vi "CODMn通讯.vi"() -> ()   [LabVIEW 2016]
uses:
  <vilib>/Plasmionique/MB Master/MB Master.lvlib
  <vilib>/Utility/config.llb/NI_LVConfig.lvlib
panel:
  in  "读取数据":bool
  in  "释放串口":bool
  in  "打开串口":bool
  out "队列中元素数量":i32
  out "元素":cluster{"命令":string}[](array[cluster])
  out "待处理插入数量":i32
  out "读取公式":u16[](array[numeric])
  out "读取参数":u16[](array[numeric])
  out "数据存储":u16[](array[numeric])
  out "温度":bool[](array[boolean])
  out "M输出点":bool[](array[boolean])
  out "ORP、时间":u16[](array[numeric])
  out "测量状态":u16[](array[numeric])
  out "通讯状态":bool
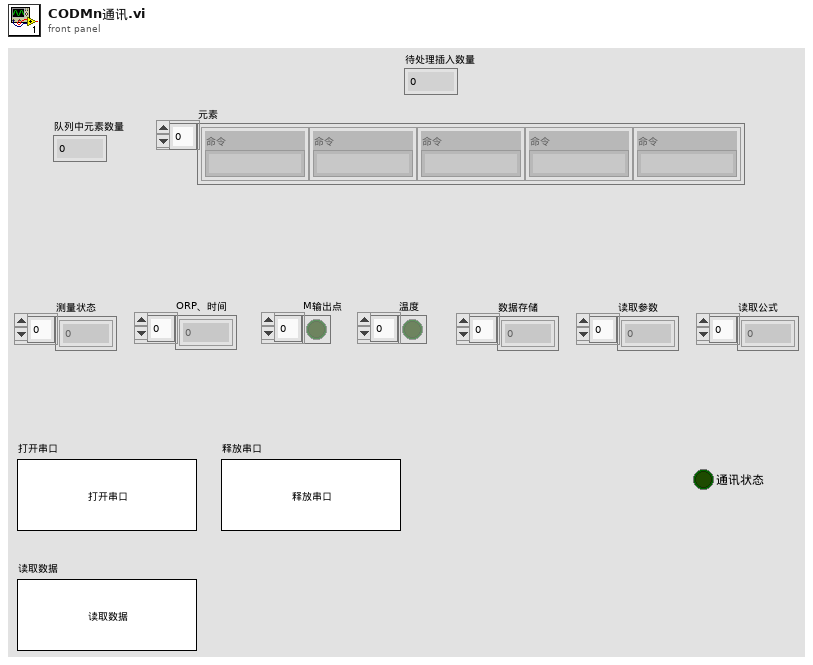
[diagram p1: front panel]
types:
  T1 = typedef "NI_LVConfig.lvlib/Config Data RefNum.ctl" = refnum<k1>
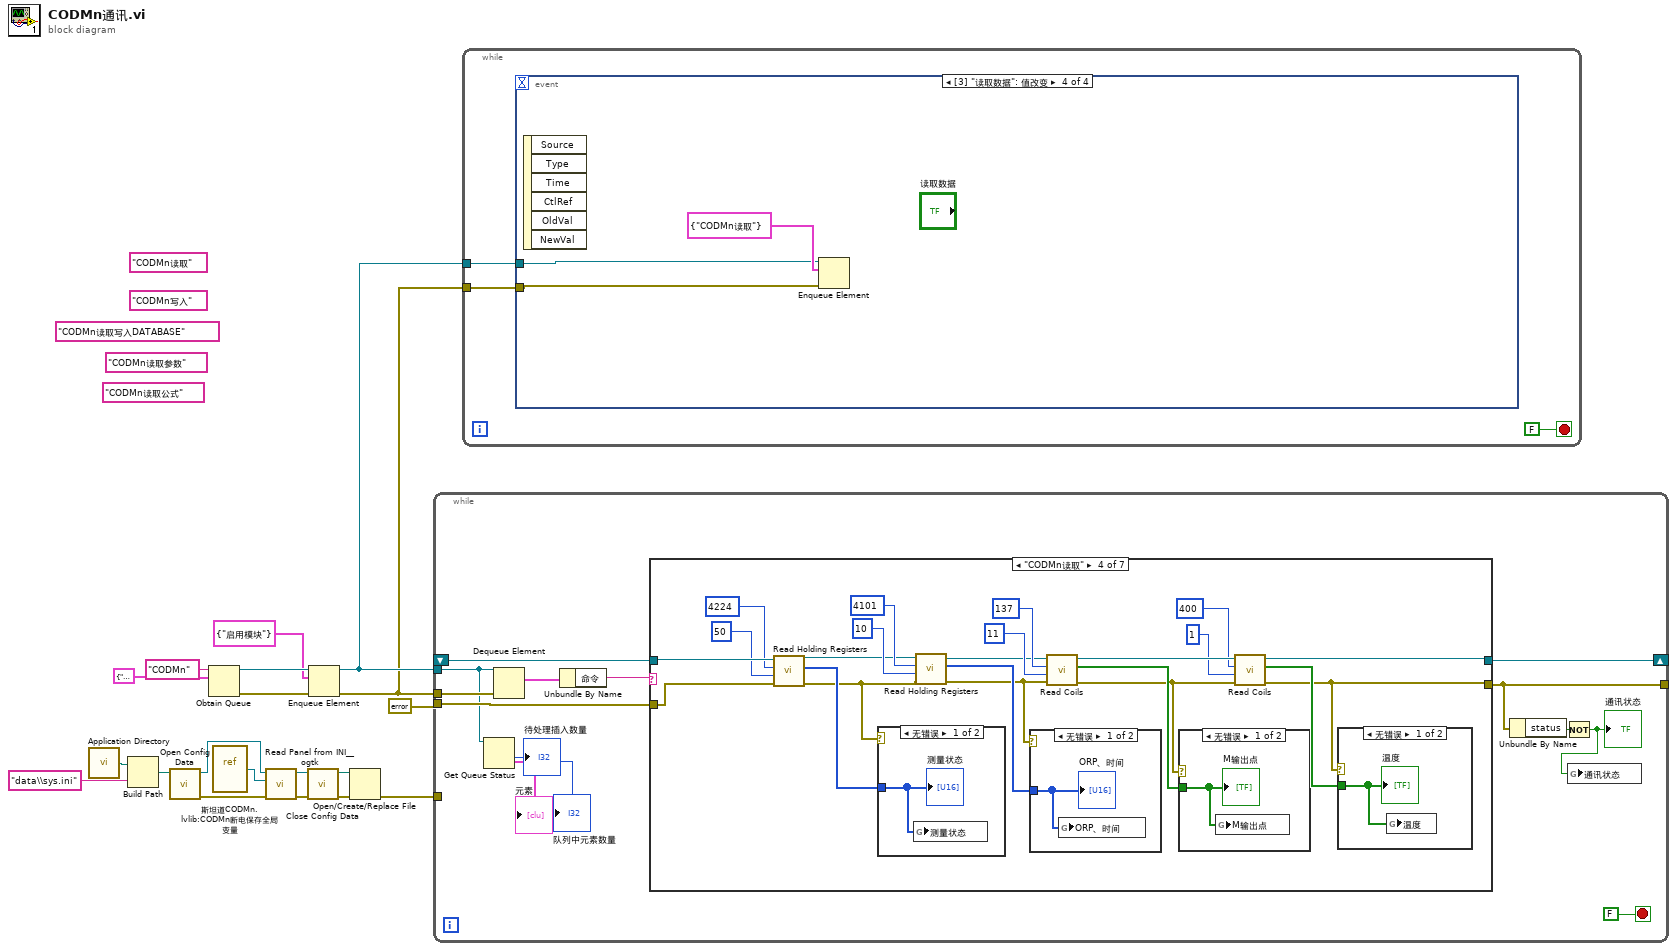
[diagram p0: block diagram]
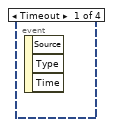
[diagram p2: hidden frame]
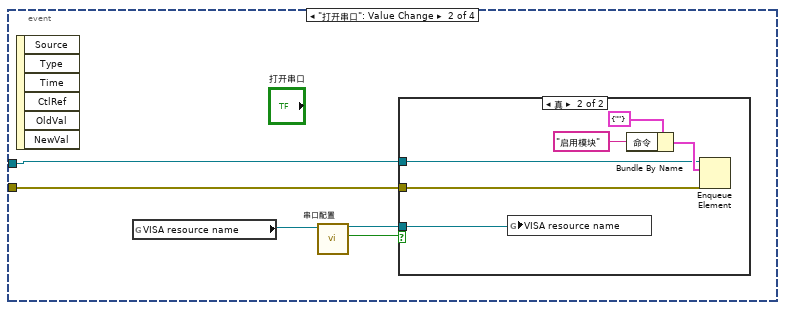
[diagram p3: hidden frame]
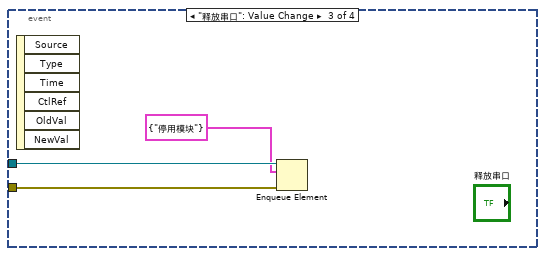
[diagram p5: hidden frame]
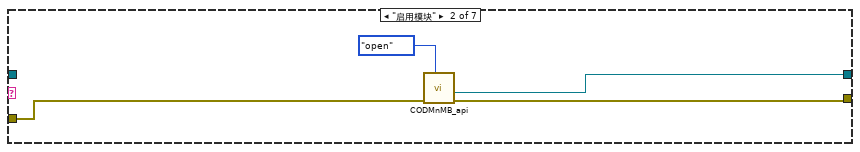
[diagram p7: hidden frame]
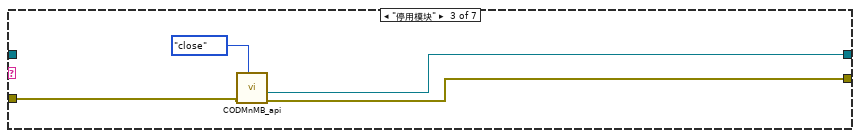
[diagram p8: hidden frame]
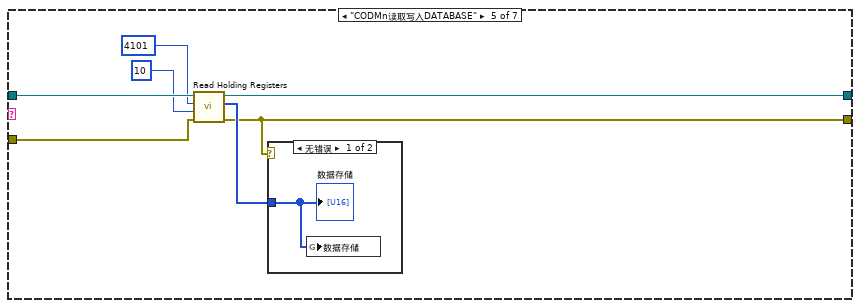
[diagram p13: hidden frame]
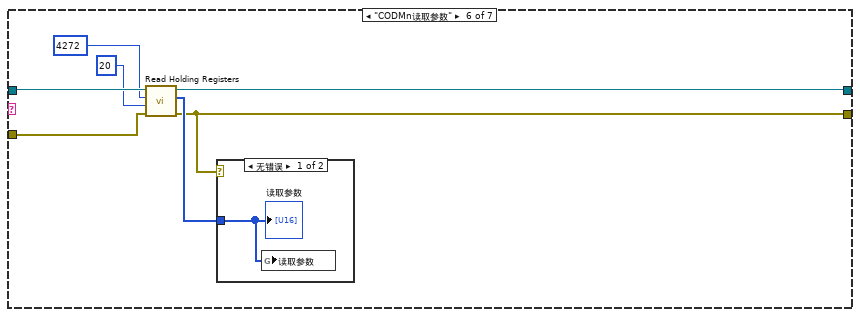
[diagram p15: hidden frame]
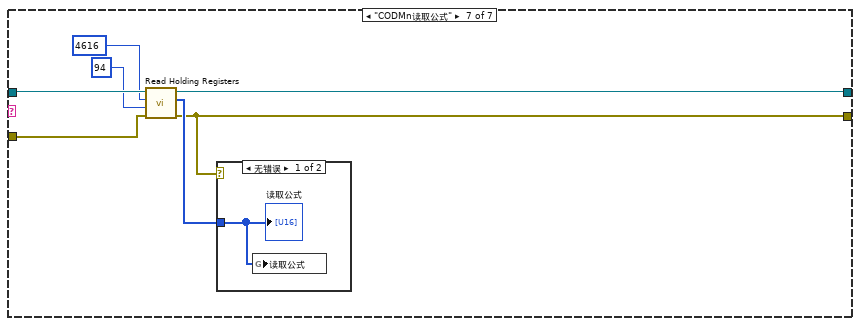
[diagram p17: hidden frame]
diagram:
  (unwired) "CODMn读取公式" ("名称（未命名）")
  (unwired) "CODMn读取写入DATABASE" ("名称（未命名）")
  (unwired) "CODMn读取参数" ("名称（未命名）")
  (unwired) "CODMn读取" ("名称（未命名）")
  (unwired) "CODMn写入" ("名称（未命名）")
  n1 = call <vilib>:"Application Directory.vi"() -> ("Application Directory"=w13:path)
  n2 = Build Path(base path=w13, name or relative path="data\\sys.ini" ("名称或相对路径")) -> (appended path=w11:path)
  n3 = call <vilib>:"Open Config Data.vi"("configuration file path"=w11) -> ("error out"=w7:errorcluster, "refnum"=w10:T1)  [unwired: 8 in, 1 out]
  n4 = Obtain Queue(name (unnamed)="CODMn" ("名称（未命名）"), element data type=cluster{"命令":string} {"命令"="启用模块"} ("元素")) -> (queue out=w16:refnum<queue>, error out=w15:errorcluster)  [unwired: 3 in, 1 out]
  n5 = vi-ref "斯坦道CODMn.lvlib:CODMn断电保存全局变量.vi"() -> (w9:refnum<vi>)
  n6 = call <userlib>:"Read Panel from INI__ogtk.vi"("error in (no error)"=w7, "VI ref"=w9, "refnum"=w10) -> ("error out"=w6:errorcluster, "refnum out"=w8:T1)  [unwired: 7 in]
  n7 = call <vilib>:"Close Config Data.vi"("error in (no error)"=w6, "refnum"=w8) -> ("error out"=w5:errorcluster, "file path"=w4:path)  [unwired: 8 in]
  n8 = Enqueue Element(queue=w16, element=cluster{"命令":string} {"命令"="启用模块"} ("元素"), error in (no error)=w15) -> (queue out=w2:refnum<queue>, error out=w1:errorcluster)  [unwired: 1 in, 1 out]
  n9 = Open/Create/Replace File(file path (use dialog)=w4, error in=w5) -> (error out=w3:errorcluster)  [unwired: 4 in, 2 out]
  n10 = while {
    tunnel: w2 -> [w23]
    tunnel: w1 -> [w32]
    tunnel: [w24] -> _
    shift-right: [w28] -> _
    shift-left: _ -> [w27]
    tunnel: errorcluster {"status"=FALSE, "code"=0, "source"=""} ("error out") -> [w26]
    tunnel: w3 -> [_]
    stop <- FALSE stop-if-true
    n11 = Get Queue Status(queue=w23) -> (# pending insert=→"待处理插入数量":i32, # elements in queue=→"队列中元素数量":i32, elements=→"元素":cluster{"命令":string}[])  [unwired: 2 in, 5 out]
    n12 = Dequeue Element(queue=w23, error in (no error)=w32) -> (element=w31:cluster{"命令":string})  [unwired: 1 in, 3 out]
    n13 = Unbundle By Name(w31) -> ("命令"=w30:string)
    n14 = case shown="\"CODMn读取\"" w30 {
      tunnel: [w35 w36 w40 w51 w72 w79 w89] -> w28
      tunnel: [w34 w39 w41 w44 w70 w78 w88] -> w24
      tunnel: w27 -> [w35 _ _ w65 w76 w84 w92]
      tunnel: w26 -> [w34 w37 w42 w64 w73 w83 w91]
      frame Default {
      }
      frame "启用模块" {
        n15 = call "CODMnMB_api.vi"("STEP"=enum16{"open", "read", "write", "close"}."open", "Error in"=w37) -> ("error out"=w39:errorcluster, "MB session out"=w36:refnum<class "MB_Master.lvclass">)  [unwired: 6 in, 2 out]
      }
      frame "停用模块" {
        n16 = call "CODMnMB_api.vi"("STEP"=enum16{"open", "read", "write", "close"}."close", "Error in"=w42) -> ("error out"=w41:errorcluster, "MB session out"=w40:refnum<class "MB_Master.lvclass">)  [unwired: 6 in, 2 out]
      }
      frame "CODMn读取" {
        n17 = call <vilib>:"Read Holding Registers.vi"("error in (no error)"=w64, "quantity"=u16 50 ("number of holding registers"), "starting address"=u16 4224, "MB session in"=w65) -> ("error out"=w55:errorcluster, "Registers"=w61:u16[], "MB session out"=w56:refnum<class "MB_Master.lvclass">)  [unwired: 5 in]
        n18 = case shown="无错误" w55 {
          tunnel: w61 -> [w69 _]
          frame No Error {
            n19 = global write "COD读取DATA全局.vi" "测量状态"(w69) -> ()
            "测量状态" <- w69
          }
          frame Error {
          }
        }
        n20 = call <vilib>:"Read Holding Registers.vi"("error in (no error)"=w55, "quantity"=u16 10, "starting address"=u16 4101, "MB session in"=w56) -> ("error out"=w50:errorcluster, "Registers"=w54:u16[], "MB session out"=w53:refnum<class "MB_Master.lvclass">)  [unwired: 5 in]
        n21 = case shown="无错误" w50 {
          tunnel: w54 -> [w68 _]
          frame No Error {
            n22 = global write "COD读取DATA全局.vi" "ORP、时间"(w68) -> ()
            "ORP、时间" <- w68
          }
          frame Error {
          }
        }
        n23 = call <vilib>:"Read Coils.vi"("error in (no error)"=w50, "quantity"=u16 11, "starting address"=u16 137, "MB session in"=w53) -> ("error out"=w48:errorcluster, "Coils"=w49:bool[], "MB session out"=w52:refnum<class "MB_Master.lvclass">)  [unwired: 5 in]
        n24 = case shown="无错误" w48 {
          tunnel: w49 -> [w67 _]
          frame No Error {
            n25 = global write "COD读取DATA全局.vi" "M输出点"(w67) -> ()
            "M输出点" <- w67
          }
          frame Error {
          }
        }
        n26 = call <vilib>:"Read Coils.vi"("error in (no error)"=w48, "quantity"=u16 1, "starting address"=u16 400, "MB session in"=w52) -> ("error out"=w44:errorcluster, "Coils"=w45:bool[], "MB session out"=w51:refnum<class "MB_Master.lvclass">)  [unwired: 5 in]
        n27 = case shown="无错误" w44 {
          tunnel: w45 -> [w66 _]
          frame No Error {
            n28 = global write "COD读取DATA全局.vi" "温度"(w66) -> ()
            "温度" <- w66
          }
          frame Error {
          }
        }
      }
      frame "CODMn读取写入DATABASE" {
        n29 = call <vilib>:"Read Holding Registers.vi"("error in (no error)"=w73, "quantity"=u16 10 ("number of holding registers"), "starting address"=u16 4101, "MB session in"=w76) -> ("error out"=w70:errorcluster, "Registers"=w71:u16[], "MB session out"=w72:refnum<class "MB_Master.lvclass">)  [unwired: 5 in]
        n30 = case shown="无错误" w70 {
          tunnel: w71 -> [w77 _]
          frame No Error {
            n31 = global write "COD读取DATA全局.vi" "数据存储"(w77) -> ()
            "数据存储" <- w77
          }
          frame Error {
          }
        }
      }
      frame "CODMn读取参数" {
        n32 = call <vilib>:"Read Holding Registers.vi"("error in (no error)"=w83, "quantity"=u16 20 ("number of holding registers"), "starting address"=u16 4272, "MB session in"=w84) -> ("error out"=w78:errorcluster, "Registers"=w80:u16[], "MB session out"=w79:refnum<class "MB_Master.lvclass">)  [unwired: 5 in]
        n33 = case shown="无错误" w78 {
          tunnel: w80 -> [w85 _]
          frame No Error {
            n34 = global write "COD读取DATA全局.vi" "读取参数"(w85) -> ()
            "读取参数" <- w85
          }
          frame Error {
          }
        }
      }
      frame "CODMn读取公式" {
        n35 = call <vilib>:"Read Holding Registers.vi"("error in (no error)"=w91, "quantity"=u16 94 ("number of holding registers"), "starting address"=u16 4616, "MB session in"=w92) -> ("error out"=w88:errorcluster, "Registers"=w90:u16[], "MB session out"=w89:refnum<class "MB_Master.lvclass">)  [unwired: 5 in]
        n36 = case shown="无错误" w88 {
          tunnel: w90 -> [w93 _]
          frame No Error {
            n37 = global write "COD读取DATA全局.vi" "读取公式"(w93) -> ()
            "读取公式" <- w93
          }
          frame Error {
          }
        }
      }
    }
    n38 = Unbundle By Name(w24) -> ("status"=w29:bool)
    n39 = Not(x=w29) -> (.not. x?=w25:bool)
    "通讯状态" <- w25
    n40 = global write "COD读取DATA全局.vi" "通讯状态"(w25) -> ()
  }
  n41 = while {
    tunnel: w2 -> [w95]
    tunnel: w1 -> [w94]
    stop <- FALSE stop-if-true
    n42 = event shown="[3] \"读取数据\": 值改变" {
      selector: _ -> [_ _ _ _]
      dyn-events: _ -> [_ _ _ _]
      timeout: _ -> [_ _ _ _]
      tunnel: w95 -> [_ w98 w110 w112]
      tunnel: w94 -> [_ w97 w109 w111]
      event Timeout {
        n43 = event-data() -> ()  [unwired: 1 in, 3 out]
      }
      event "打开串口": Value Change {
        n44 = event-data() -> ()  [unwired: 1 in, 6 out]
        n45 = global read "CODMn断电保存全局变量.vi" "VISA resource name"() -> (w101:refnum<visa-resource-name>)
        n46 = call "串口配置.vi"("VISA资源名称"=w101) -> ("确认 2"=w99:bool, "VISA资源名称 2"=w100:refnum<visa-resource-name>)  [unwired: 9 in]
        n47 = case shown="真" w99 {
          tunnel: w100 -> [_ w107]
          tunnel: w98 -> [_ w103]
          tunnel: w97 -> [_ w102]
          frame False {
          }
          frame True {
            n48 = global write "CODMn断电保存全局变量.vi" "VISA resource name"(w107) -> ()
            n49 = Bundle By Name(cluster=cluster{"命令":string} {"命令"=""} ("元素"), "命令"="启用模块" ("名称（未命名）")) -> (w104:cluster{"命令":string})
            n50 = Enqueue Element(queue=w103, element=w104, error in (no error)=w102) -> ()  [unwired: 1 in, 3 out]
          }
        }
      }
      event "释放串口": Value Change {
        n51 = event-data() -> ()  [unwired: 1 in, 6 out]
        n52 = Enqueue Element(queue=w110, element=cluster{"命令":string} {"命令"="停用模块"} ("元素"), error in (no error)=w109) -> ()  [unwired: 1 in, 3 out]
      }
      event "读取数据": Value Change {
        n53 = event-data() -> ()  [unwired: 1 in, 6 out]
        n54 = Enqueue Element(queue=w112, element=cluster{"命令":string} {"命令"="CODMn读取"} ("元素"), error in (no error)=w111) -> ()  [unwired: 1 in, 3 out]
      }
    }
  }
